vi "Read Configuration Parameters.vi"(8 "error in (no error)":errorcluster, 10 "refnum":T1, 11 "Example Configuration Dialog in":refnum<class "Controller Configuration.lvclass">) -> (0 "error out":errorcluster, 2 "refnum out":T1, 3 "Example Configuration Dialog out":refnum<class "Controller Configuration.lvclass">)   [LabVIEW 2016, in "Fcn Configuration.lvlib" / "Controller Configuration.lvclass"]
uses:
  <userlib>/Common Components/FCN Configuration/Controller Configuration.lvclass
  <vilib>/Utility/config.llb/Config Data RefNum.ctl
  <userlib>/Common Components/FCN Configuration/Controller Configuration.lvclass/Controller Configuration.ctl
  <userlib>/Configuration Dialog Actor/Configuration.lvclass
  <userlib>/Common Components/Common/Common.lvlib
  <vilib>/Utility/config.llb/NI_LVConfig.lvlib
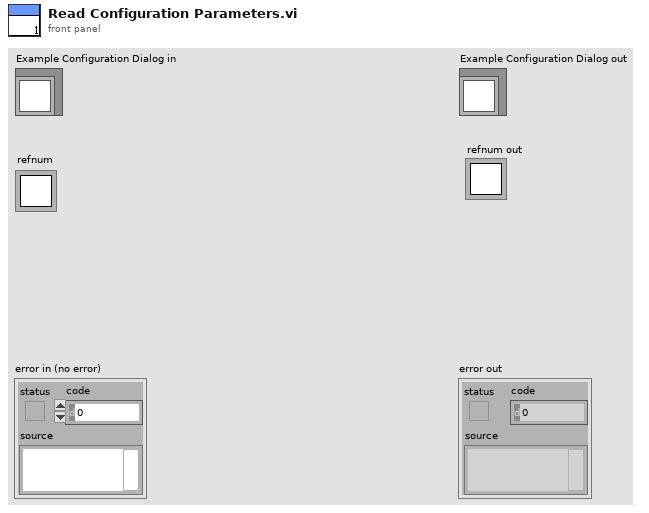
[diagram p1: front panel]
types:
  T1 = typedef "NI_LVConfig.lvlib/Config Data RefNum.ctl" = refnum<k1>
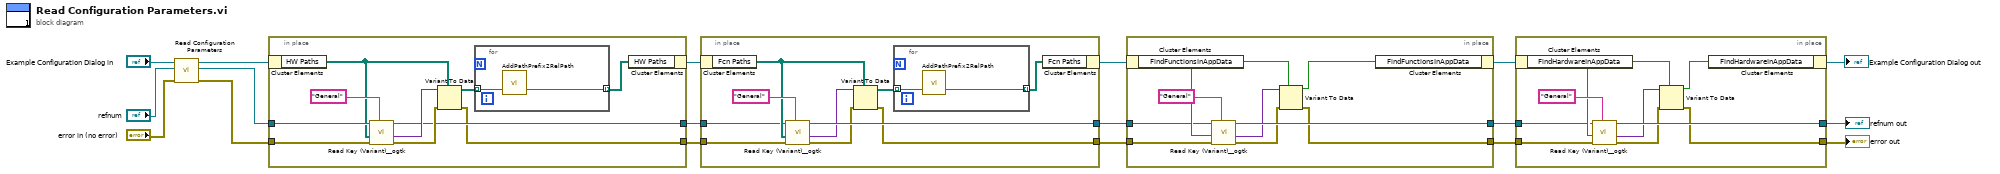
[diagram p0: block diagram]
diagram:
  n1 = call-parent "Read Configuration Parameters.vi"("error in (no error)"="error in (no error)", "refnum"="refnum", "Configuration in"="Example Configuration Dialog in") -> ("error out"=w14:errorcluster, "refnum out"=w15:T1, "Configuration out"=w13:refnum<class "Controller Configuration.lvclass">)  [unwired: 6 in]
  n2 = in-place "In Place Element Structure" {
    in-place-border: w15 -> [w26]
    in-place-border: w14 -> [w21]
    in-place-border: [w24] -> w11
    in-place-border: [w23] -> w10
    n3 = in-place-cluster #1(w13) -> ("HW Paths"=w22:path[])
    n4 = call <userlib>:"Read Key (Variant)__ogtk.vi"("section"="General", "error in (no error)"=w21, "type"=w22, "refnum"=w26) -> ("error out"=w27:errorcluster, "key-value"=w28:variant, "refnum out"=w24:T1)  [unwired: 4 in, 1 out]
    n5 = Variant To Data(error in=w27, type=w22, Variant=w28) -> (data=w20:path[], error out=w23:errorcluster)
    n6 = for {
      tunnel: w20 -> [w30] mode=indexing
      tunnel: [w29] -> w19 mode=indexing
      n7 = call <userlib>:"AddPathPrefix2RelPath.vi"("Path"=w30) -> ("Path out"=w29:path)  [unwired: 1 in, 1 out]
    }
    n8 = in-place-cluster #1("HW Paths"=w19) -> (w12:refnum<class "Controller Configuration.lvclass">)
  }
  n9 = in-place "In Place Element Structure" {
    in-place-border: [w35] -> w4
    in-place-border: [w39] -> w5
    in-place-border: w11 -> [w34]
    in-place-border: w10 -> [w33]
    n10 = in-place-cluster #2(w12) -> ("Fcn Paths"=w38:path[])
    n11 = call <userlib>:"Read Key (Variant)__ogtk.vi"("section"="General", "error in (no error)"=w33, "type"=w38, "refnum"=w34) -> ("error out"=w36:errorcluster, "key-value"=w37:variant, "refnum out"=w39:T1)  [unwired: 4 in, 1 out]
    n12 = Variant To Data(error in=w36, type=w38, Variant=w37) -> (data=w32:path[], error out=w35:errorcluster)
    n13 = for {
      tunnel: w32 -> [w42] mode=indexing
      tunnel: [w41] -> w31 mode=indexing
      n14 = call <userlib>:"AddPathPrefix2RelPath.vi"("Path"=w42) -> ("Path out"=w41:path)  [unwired: 1 in, 1 out]
    }
    n15 = in-place-cluster #2("Fcn Paths"=w31) -> (w6:refnum<class "Controller Configuration.lvclass">)
  }
  n16 = in-place "In Place Element Structure" {
    in-place-border: [w45] -> w8
    in-place-border: [w50] -> w9
    in-place-border: w5 -> [w44]
    in-place-border: w4 -> [w43]
    n17 = in-place-cluster #3(w6) -> ("FindFunctionsInAppData"=w49:bool)
    n18 = call <userlib>:"Read Key (Variant)__ogtk.vi"("section"="General", "error in (no error)"=w43, "type"=w49, "refnum"=w44) -> ("error out"=w46:errorcluster, "key-value"=w48:variant, "refnum out"=w50:T1)  [unwired: 4 in, 1 out]
    n19 = Variant To Data(error in=w46, type=w49, Variant=w48) -> (data=w47:bool, error out=w45:errorcluster)
    n20 = in-place-cluster #3("FindFunctionsInAppData"=w47) -> (w7:refnum<class "Controller Configuration.lvclass">)
  }
  n21 = in-place "In Place Element Structure" {
    in-place-border: [w54] -> w1
    in-place-border: [w59] -> w2
    in-place-border: w9 -> [w53]
    in-place-border: w8 -> [w52]
    n22 = in-place-cluster #4(w7) -> ("FindHardwareInAppData"=w58:bool)
    n23 = call <userlib>:"Read Key (Variant)__ogtk.vi"("section"="General", "error in (no error)"=w52, "type"=w58, "refnum"=w53) -> ("error out"=w55:errorcluster, "key-value"=w57:variant, "refnum out"=w59:T1)  [unwired: 4 in, 1 out]
    n24 = Variant To Data(error in=w55, type=w58, Variant=w57) -> (data=w56:bool, error out=w54:errorcluster)
    n25 = in-place-cluster #4("FindHardwareInAppData"=w56) -> (→"Example Configuration Dialog out":refnum<class "Controller Configuration.lvclass">)
  }
  "error out" <- w1
  "refnum out" <- w2
